vi "FRCts20_Backend_Test_Comment.vi"() -> ()   [LabVIEW 2014, in "FRCts20_Backend_TestCode.lvlib"]
uses:
  FRCts20_Backend_TestCode.lvlib
  FRCts20_Backend_API/FRCts20_Backend_API_Command_App.ctl
  FRCts20_Backend_API/FRCts20_Backend_API_Note.ctl
  FRCts20_Backend_API/FRCts20_Backend_API_Application.vi
  FRCts20_Backend_Engine.lvlib
  FRCts20_Backend_API/FRCts20_Backend_API.lvlib
panel:
  out "Get Pass/Fail":bool
  out "error out":errorcluster
  out "Del Pass/Fail":bool
  out "GetDel":u32
  out "Del":u32
  out "GetPut":u32
  out "Put":u32
  out "Put Pass/Fail":bool
  out "Post Pass/Fail":bool
  out "GetPost":u32
  out "post":u32
  out "Get":u32
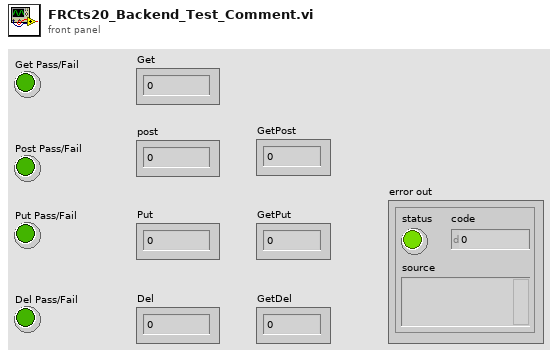
[diagram p1: front panel]
types:
  T1 = typedef "FRCts20_Backend_API.lvlib/FRCts20_Backend_API_Note.ctl" = cluster{"Note Index":u32, "Request Index":u32, "Author":string, "Time Entered":timestamp, "Text":string, "Solution":bool, "APIReturn":string}
  T2 = typedef "FRCts20_Backend_API.lvlib/FRCts20_Backend_API_Command_App.ctl" = string
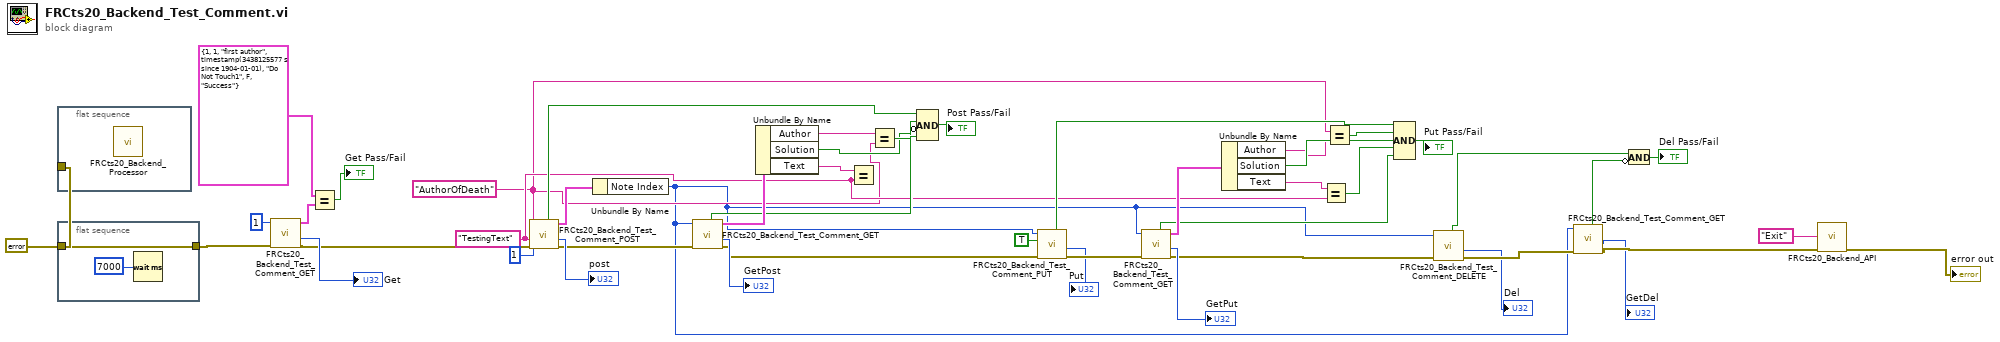
[diagram p0: block diagram]
diagram:
  w12 = "AuthorOfDeath" ("Author")
  w13 = "TestingText" ("Text")
  w48 = errorcluster {"status"=FALSE, "code"=0, "source"=""} ("error constant")
  n1 = flat-sequence {
    tunnel: w48 -> [_]
    frame #0 {
      n2 = call "FRCts20_Backend_Processor.vi"() -> ()  [unwired: 12 in]
    }
  }
  n3 = flat-sequence {
    tunnel: w48 -> [w49]
    tunnel: [w49] -> w42
    frame #0 {
      n4 = Wait (ms)(milliseconds to wait=u32 7000) -> ()  [unwired: 1 out]
    }
  }
  n5 = call "FRCts20_Backend_Test_Comment_GET.vi"("error in (no error)"=w42, "Note Index"=u32 1) -> ("error out"=w39:errorcluster, "Time (ms)"=→"Get":u32, "Note Out"=w11:T1)  [unwired: 5 in, 2 out]
  n6 = Equal?(x=T1 {"Note Index"=1, "Request Index"=1, "Author"="first author", "Time Entered"=timestamp(3438125577 s since 1904-01-01), "Text"="Do Not Touch1", "Solution"=FALSE, "APIReturn"="Success"} ("Note Out"), y=w11) -> (x = y?=→"Get Pass/Fail":bool)
  n7 = call "FRCts20_Backend_Test_Comment_POST.vi"("error in (no error)"=w39, "Text"=w13, "Author"=w12, "Req Index"=u32 1) -> ("error out"=w36:errorcluster, "Time (ms)"=→"post":u32, "Note Out"=w37:T1, "Success"=w33:bool)  [unwired: 3 in, 1 out]
  n8 = Unbundle By Name(w37) -> ("Note Index"=w2:u32)
  n9 = call "FRCts20_Backend_Test_Comment_GET.vi"("error in (no error)"=w36, "Note Index"=w2) -> ("error out"=w21:errorcluster, "Time (ms)"=→"GetPost":u32, "Note Out"=w35:T1, "Success"=w32:bool)  [unwired: 5 in, 1 out]
  n10 = Unbundle By Name(w35) -> ("Author"=w29:string, "Solution"=w27:bool, "Text"=w34:string)
  n11 = Equal?(x=w34, y=w13) -> ()  [unwired: 1 out]
  n12 = Equal?(x=w29, y=w12) -> (x = y?=w28:bool)
  n13 = Compound Arithmetic op=AND(w33, w28, invert w27, w32) -> (→"Post Pass/Fail":bool)
  n14 = call "FRCts20_Backend_Test_Comment_PUT.vi"("error in (no error)"=w21, "Solution"=TRUE, "Note Index"=w2) -> ("error out"=w23:errorcluster, "Time (ms)"=→"Put":u32, "Success"=w26:bool)  [unwired: 4 in, 2 out]
  n15 = call "FRCts20_Backend_Test_Comment_GET.vi"("error in (no error)"=w23, "Note Index"=w2) -> ("error out"=w3:errorcluster, "Time (ms)"=→"GetPut":u32, "Note Out"=w25:T1, "Success"=w18:bool)  [unwired: 5 in, 1 out]
  n16 = Unbundle By Name(w25) -> ("Author"=w16:string, "Solution"=w19:bool, "Text"=w17:string)
  n17 = Equal?(x=w17, y=w13) -> (x = y?=w14:bool)
  n18 = Equal?(x=w12, y=w16) -> (x = y?=w15:bool)
  n19 = Compound Arithmetic op=AND(w26, w15, w19, w14, w18) -> (→"Put Pass/Fail":bool)
  n20 = call "FRCts20_Backend_Test_Comment_DELETE.vi"("error in (no error)"=w3, "Com Indx"=w2) -> ("error out"=w6:errorcluster, "Time (ms)"=→"Del":u32, "Success"=w5:bool)  [unwired: 5 in, 2 out]
  n21 = call "FRCts20_Backend_Test_Comment_GET.vi"("error in (no error)"=w6, "Note Index"=w2) -> ("error out"=w8:errorcluster, "Time (ms)"=→"GetDel":u32, "Success"=w9:bool)  [unwired: 5 in, 2 out]
  n22 = Compound Arithmetic op=AND(w5, invert w9) -> (→"Del Pass/Fail":bool)
  n23 = call-poly "FRCts20_Backend_API.vi"("error in (no error)"=w8, "Command"=T2 "Exit") -> ("error out"=→"error out":errorcluster)  [unwired: 7 in, 2 out]
